vi "TcA02-001_ReadingLockingAndSettingAnObjectsAttributes.vi"(1 "Input buffer":T3="1", 3 "Invocation info":T2, 5 "error in (no error)":errorcluster, 6 "Add log to result?":bool) -> (16 "Test Data":T1 {"Numeric Measurement" format="%.2f"}, 19 "error out":errorcluster)   [LabVIEW 2009]
doc: "Test case template."
uses:
  Shared/Support_InputBuffer.ctl
  Shared/Support_InvocationInfo.ctl
  Shared/Support_TestData.ctl
  TestClasses/G#SubSubClass2_class/G#SubSubClass2.lvclass
  TestClasses/G#SubClass2_class/G#SubClass2.lvclass
  TestClasses/G#BaseClass2_class/G#BaseClass2.lvclass
  <vilib>/addons/_AddQ/G#Object/G#Object.lvclass
panel:
  in  "Test name":string="TcA02-001 Reading, locking and setting an objects attributes"
  out "Test result":bool
  out "Result":string
  # "Verify that an object be locked, read and\nset the attributes and thereby unlock them."
  # "Sub test case"
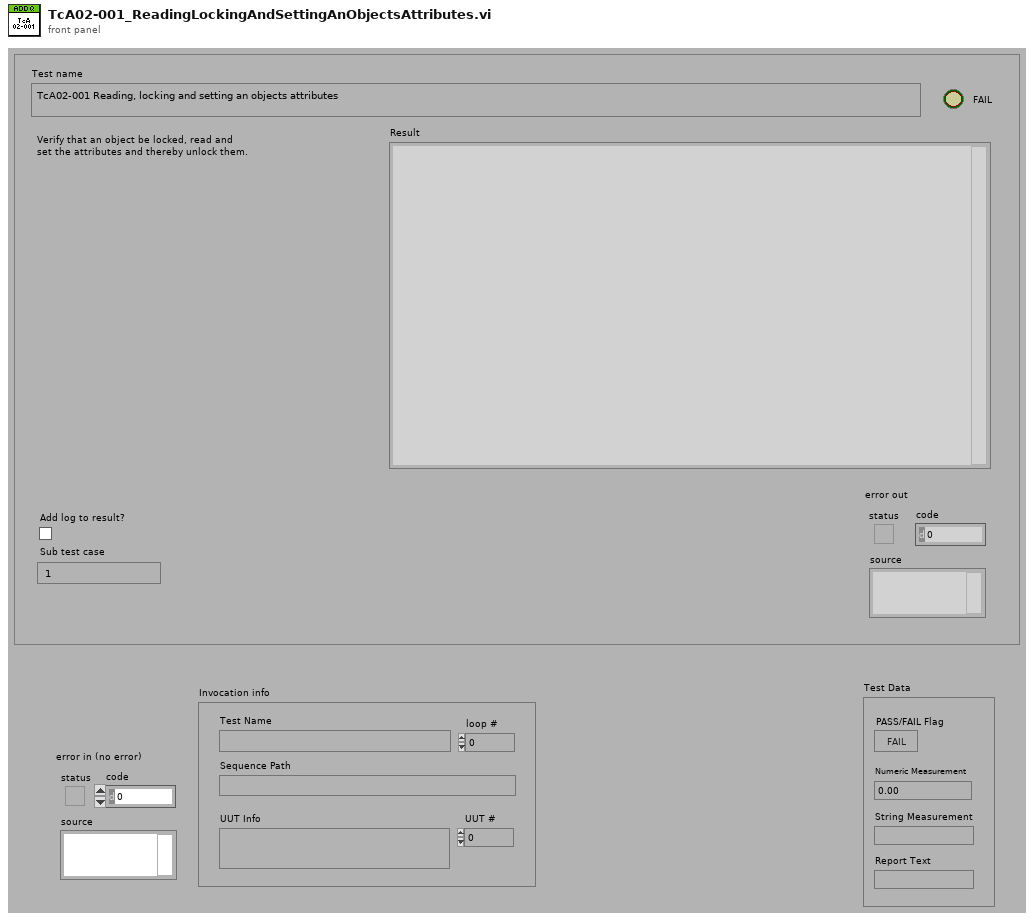
[diagram p1: front panel]
types:
  T1 = typedef "Support_TestData.ctl" = cluster{"PASS/FAIL Flag":bool, "Numeric Measurement":dbl, "String Measurement":string, "Report Text":string}
  T2 = typedef "Support_InvocationInfo.ctl" = cluster{"UUT #":i32, "loop #":i32, "UUT Info":string, "Test Name":string, "Sequence Path":path}
  T3 = typedef "Support_InputBuffer.ctl" = string
  T4 = typedef "Support_ResultType.ctl" = cluster{"Pass":bool, "Comment":string, "MeasurementValue":dbl}
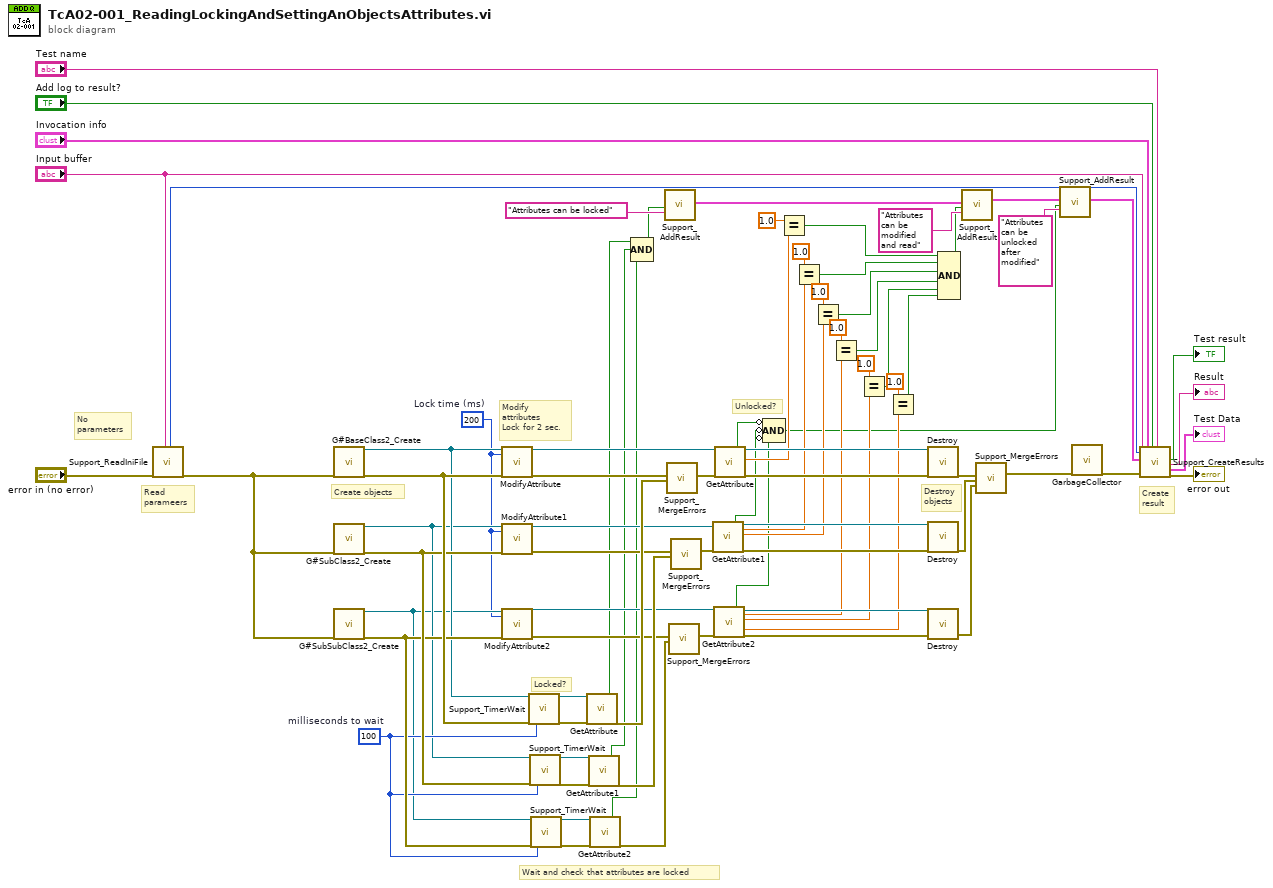
[diagram p0: block diagram]
diagram:
  w59 = u32 100  # milliseconds to wait
  w3 = u32 200  # Lock time (ms)
  # "Locked?"
  # "Unlocked?"
  # "Destroy\nobjects"
  # "Create objects"
  # "Modify\nattributes\nLock for 2 sec."
  # "Wait and check that attributes are locked"
  # "No\nparameters"
  # "Create\nresult"
  # "Read\nparameers"
  n1 = call "Support_ReadIniFile.vi"("error in (no error)"="error in (no error)", "Sub test case"="Input buffer") -> ("Timer start"=w69:u32, "error out"=w68:errorcluster)  [unwired: 10 in, 6 out]
  n2 = call "G#BaseClass2_Create.vi"("error in (no error)"=w68) -> ("reference out"=w56:refnum<class "G#BaseClass2.lvclass">, "error out"=w67:errorcluster)  [unwired: 17 in]
  n3 = call "G#SubClass2_Create.vi"("error in (no error)"=w68) -> ("reference out"=w54:refnum<class "G#SubClass2.lvclass">, "error out"=w66:errorcluster)  [unwired: 17 in]
  n4 = call "G#SubSubClass2_Create.vi"("error in (no error)"=w68) -> ("reference out"=w50:refnum<class "G#SubSubClass2.lvclass">, "error out"=w65:errorcluster)  [unwired: 17 in]
  n5 = call-dynamic "ModifyAttribute.vi"("reference in"=w56, "Lock time (ms)"=w3, "error in (no error)"=w67) -> ("reference out"=w40:refnum<class "G#BaseClass2.lvclass">, "error out"=w49:errorcluster)  [unwired: 14 in, 1 out]
  n6 = call-dynamic "ModifyAttribute1.vi"("reference in"=w54, "Lock time (ms)"=w3, "error in (no error)"=w66) -> ("reference out"=w38:refnum<class "G#SubClass2.lvclass">, "error out"=w48:errorcluster)  [unwired: 14 in, 1 out]
  n7 = call-dynamic "ModifyAttribute2.vi"("reference in"=w50, "Lock time (ms)"=w3, "error in (no error)"=w65) -> ("reference out"=w36:refnum<class "G#SubSubClass2.lvclass">, "error out"=w47:errorcluster)  [unwired: 14 in, 1 out]
  n8 = call "Support_TimerWait.vi"("error in (no error)"=w67, "milliseconds to wait"=w59) -> ("error out"=w57:errorcluster)  [unwired: 17 in]
  n9 = call "Support_TimerWait.vi"("error in (no error)"=w66, "milliseconds to wait"=w59) -> ("error out"=w53:errorcluster)  [unwired: 17 in]
  n10 = call "Support_TimerWait.vi"("error in (no error)"=w65, "milliseconds to wait"=w59) -> ("error out"=w51:errorcluster)  [unwired: 17 in]
  n11 = call-dynamic "GetAttribute.vi"("reference in"=w56, "error in (no error)"=w57) -> ("Locked"=w34:bool, "error out"=w58:errorcluster)  [unwired: 13 in, 3 out]
  n12 = call-dynamic "GetAttribute1.vi"("reference in"=w54, "error in (no error)"=w53) -> ("Locked"=w2:bool, "error out"=w55:errorcluster)  [unwired: 12 in, 4 out]
  n13 = call-dynamic "GetAttribute2.vi"("reference in"=w50, "error in (no error)"=w51) -> ("Locked"=w1:bool, "error out"=w52:errorcluster)  [unwired: 11 in, 5 out]
  n14 = Compound Arithmetic op=AND(w34, w2, w1) -> (w31:bool)
  n15 = call "Support_AddResult.vi"("Pass"=w31, "Comment"="Attributes can be locked") -> ("Results out"=w32:T4[])  [unwired: 17 in]
  n16 = call "Support_MergeErrors.vi"("error in 1"=w49, "error in 2"=w58) -> ("error out"=w46:errorcluster)  [unwired: 16 in, 1 out]
  n17 = call "Support_MergeErrors.vi"("error in 1"=w47, "error in 2"=w52) -> ("error out"=w44:errorcluster)  [unwired: 16 in, 1 out]
  n18 = call "Support_MergeErrors.vi"("error in 1"=w48, "error in 2"=w55) -> ("error out"=w42:errorcluster)  [unwired: 16 in, 1 out]
  n19 = call-dynamic "GetAttribute1.vi"("reference in"=w38, "error in (no error)"=w42) -> ("Locked"=w5:bool, "reference out"=w37:refnum<class "G#SubClass2.lvclass">, "Base class.Numeric"=w26:dbl, "SubAttribute"=w24:dbl, "error out"=w41:errorcluster)  [unwired: 12 in, 1 out]
  n20 = call-dynamic "GetAttribute2.vi"("reference in"=w36, "error in (no error)"=w44) -> ("Locked"=w4:bool, "reference out"=w35:refnum<class "G#SubSubClass2.lvclass">, "Base class.Base class.Numeric"=w22:dbl, "Base class.SubAttribute"=w19:dbl, "SubSubAttribute"=w18:dbl, "error out"=w43:errorcluster)  [unwired: 11 in, 1 out]
  n21 = call-dynamic "GetAttribute.vi"("reference in"=w40, "error in (no error)"=w46) -> ("Locked"=w6:bool, "reference out"=w39:refnum<class "G#BaseClass2.lvclass">, "Numeric"=w29:dbl, "error out"=w45:errorcluster)  [unwired: 13 in, 1 out]
  n22 = Compound Arithmetic op=AND(invert w6, invert w5, invert w4) -> (w7:bool)
  n23 = Equal?(x=1.0, y=w29) -> (x = y?=w17:bool)
  n24 = Equal?(x=1.0, y=w26) -> (x = y?=w16:bool)
  n25 = Equal?(x=1.0, y=w24) -> (x = y?=w15:bool)
  n26 = Equal?(x=1.0, y=w22) -> (x = y?=w14:bool)
  n27 = Equal?(x=1.0, y=w19) -> (x = y?=w13:bool)
  n28 = Equal?(x=1.0, y=w18) -> (x = y?=w12:bool)
  n29 = call-dynamic "Destroy.vi"("reference in"=w39, "error in (no error)"=w45) -> ("error out"=w64:errorcluster)  [unwired: 16 in, 1 out]
  n30 = call-dynamic "Destroy.vi"("reference in"=w37, "error in (no error)"=w41) -> ("error out"=w63:errorcluster)  [unwired: 16 in, 1 out]
  n31 = call-dynamic "Destroy.vi"("reference in"=w35, "error in (no error)"=w43) -> ("error out"=w62:errorcluster)  [unwired: 16 in, 1 out]
  n32 = Compound Arithmetic op=AND(w17, w16, w15, w14, w13, w12) -> (w11:bool)
  n33 = call "Support_AddResult.vi"("Results in"=w32, "Pass"=w11, "Comment"="Attributes can be modified and read") -> ("Results out"=w10:T4[])  [unwired: 16 in]
  n34 = call "Support_MergeErrors.vi"("error in 1"=w64, "error in 2"=w63, "error in 3"=w62) -> ("error out"=w61:errorcluster)  [unwired: 15 in, 1 out]
  n35 = call "Support_AddResult.vi"("Results in"=w10, "Pass"=w7, "Comment"="Attributes can be unlocked after modified") -> ("Results out"=w9:T4[])  [unwired: 16 in]
  n36 = call <vilib>:"GarbageCollector.vi"("error in (no error)"=w61) -> ("error out"=w60:errorcluster)  [unwired: 16 in, 2 out]
  n37 = call "Support_CreateResults.vi"("Sub test case"="Input buffer", "Timer start"=w69, "Results"=w9, "error in (no error)"=w60, "Invocation info"="Invocation info", "Add log to result?"="Add log to result?", "Test name"="Test name") -> ("Pass/fail flag"=→"Test result":bool, "Result"=→"Result":string, "Test Data"=→"Test Data":T1, "error out"=→"error out":errorcluster)  [unwired: 9 in]
